vi "Dipper Fridge Resistance Measurement 1.2.vi"() -> ()   [LabVIEW 2011]
uses:
  <vilib>/express/express arith-compare/Formula/XNode/ExpressFormulaBlockNode.xnode
panel:
  in  "Timer":bool caption="Reset"
  out "Time Elapsed":string
  out "Output Power":dbl[unit]
  out "Heater Power (%)":string
  in  "Save":bool
  out "var":i32
  in  "error in (no error) 2":errorcluster
  in  "Output Range":string(combo)
  in  "Heater Power (%)":dbl caption="y"
  out "Heater Type (in Ohm)":string
  out "Heater Current (in %)":string
  out "Heater":bool
  in  "Heater":bool
  out "Boolean":bool
  in  "Power":bool
  in  "Date format (0)":enum16{"short", "long", "abbreviated"}(ring)
  out "Sample (Lakeshore)":cluster{dbl[], dbl[unit][]}(graph)
  out "Thermometer A":cluster{dbl[], dbl[unit][]}(graph)
  out "size (in bytes)":i64
  out "Thermometer (Ge17035)":cluster{dbl[], dbl[]}(graph)
  out "Warning":string="Can't be smaller than 1 s"
  in  "File Path":path
  out "current time":timestamp
  out "Number of Data points":i32
  in  "Time delay":u32=500 min=500 max=10000
  in  "error in (no error)":errorcluster
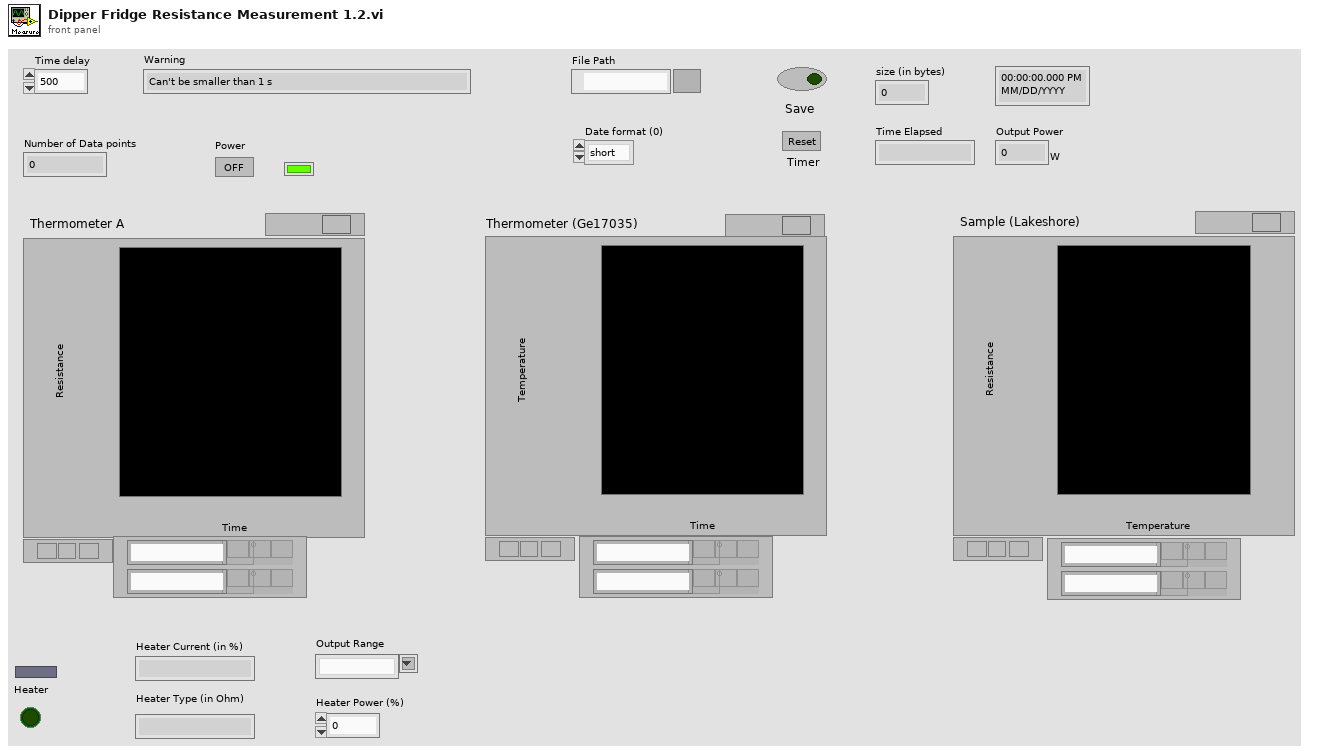
[diagram p1: front panel]
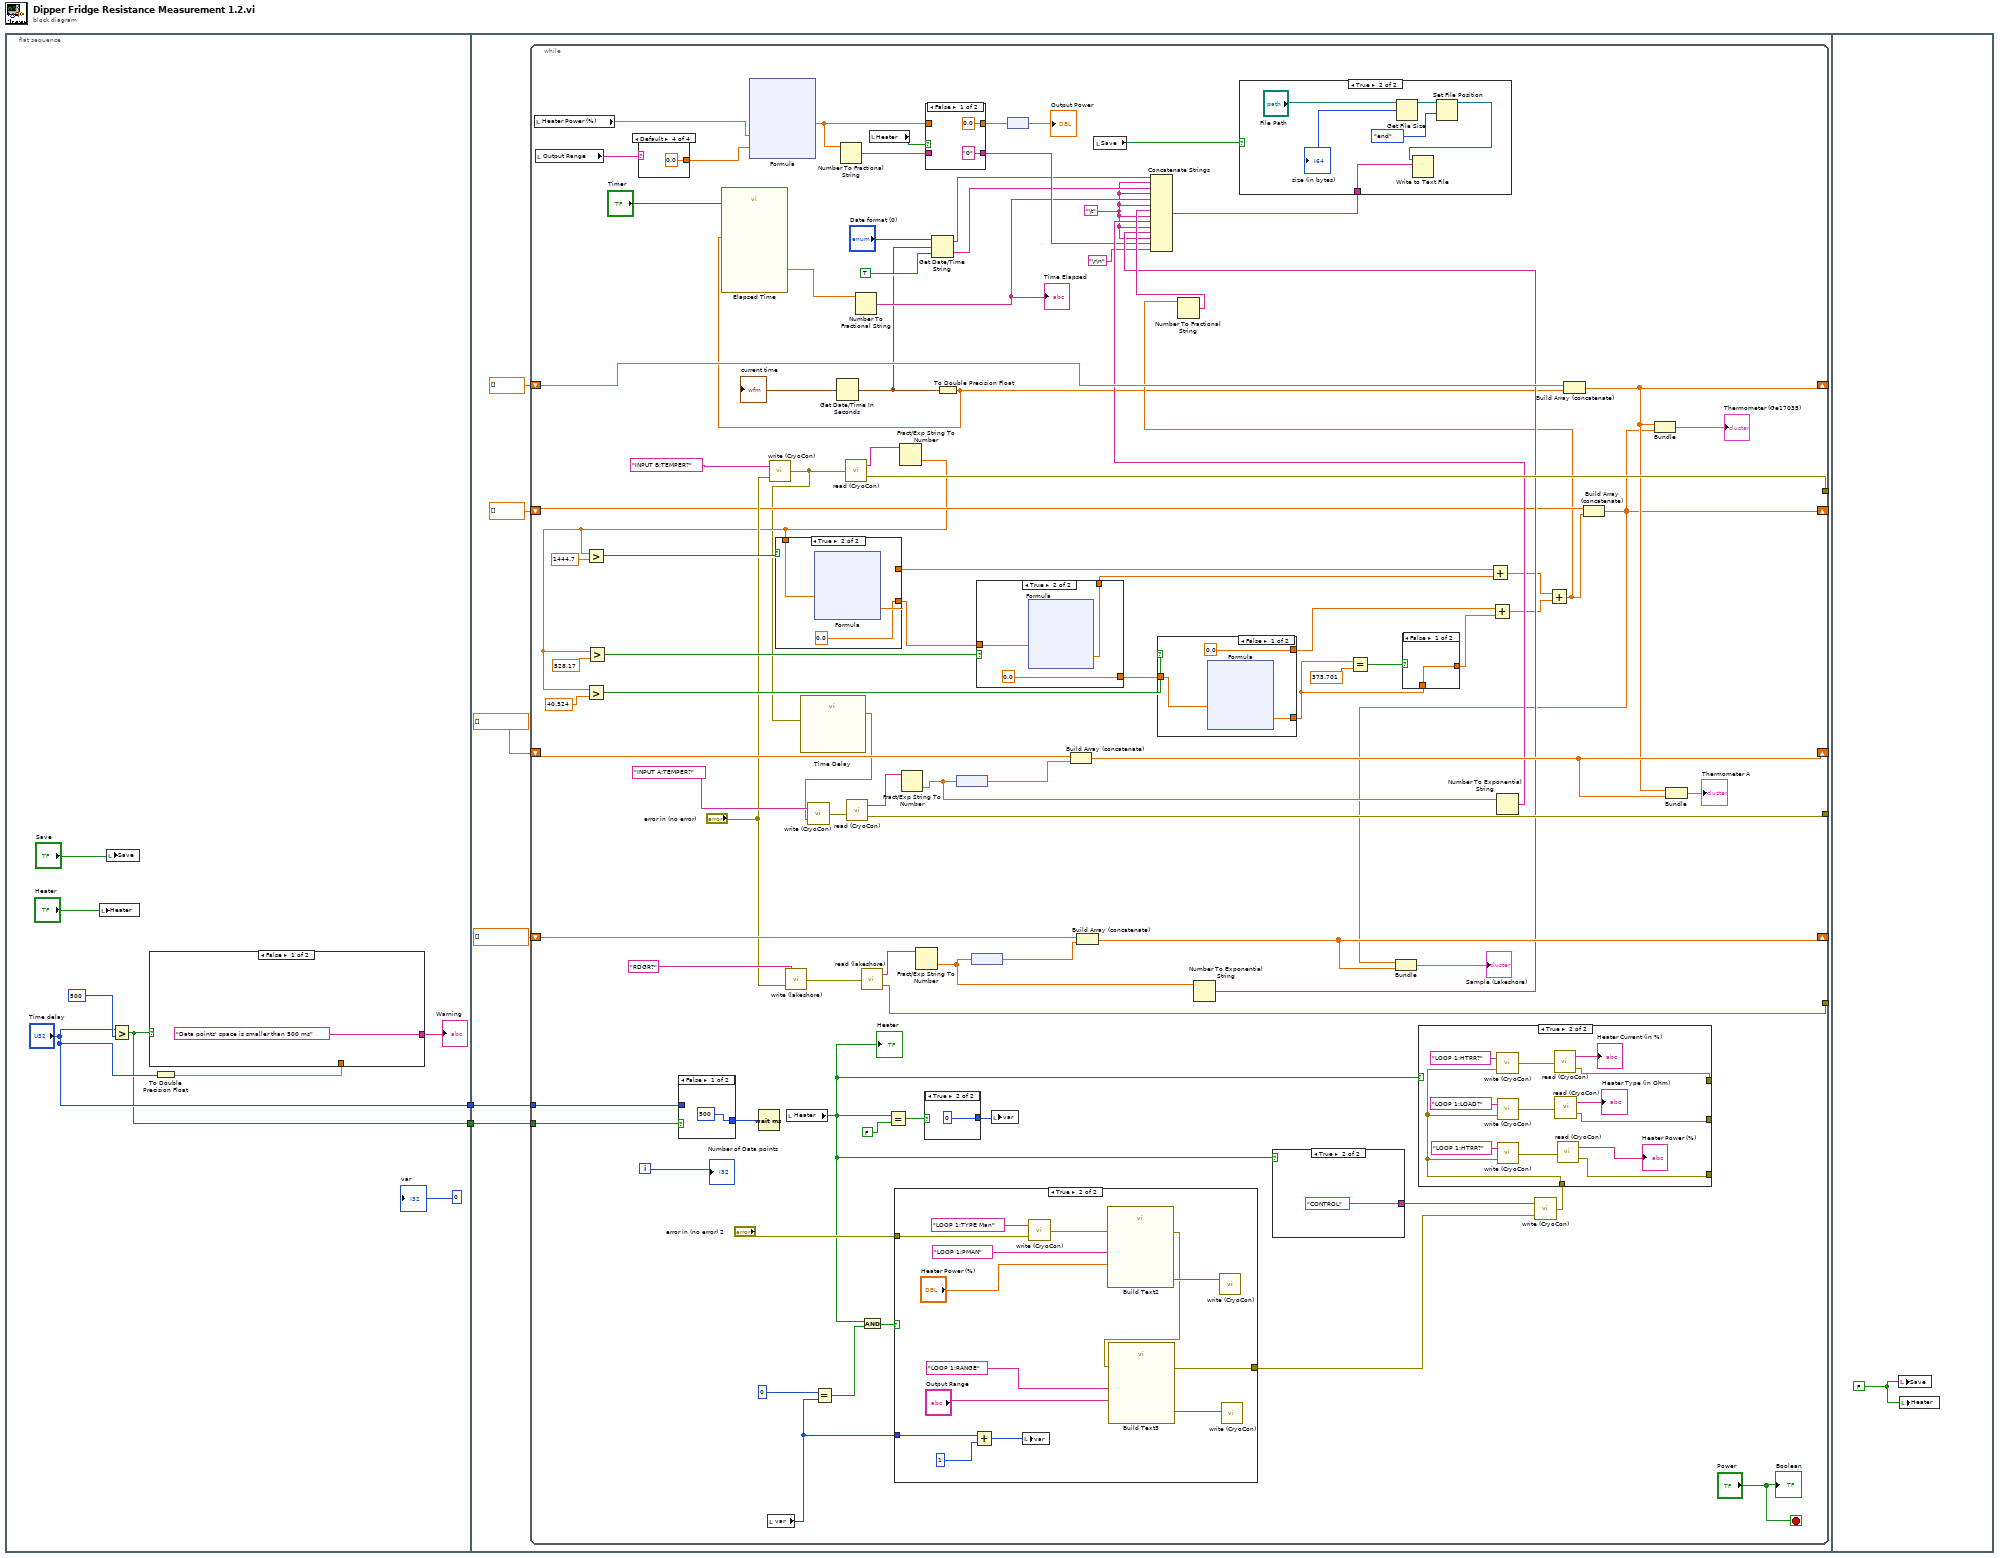
[diagram p0: block diagram]
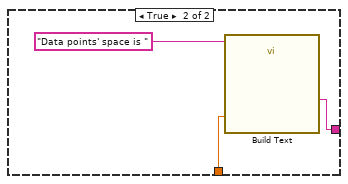
[diagram p2: hidden frame]
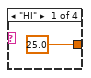
[diagram p4: hidden frame]
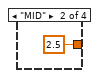
[diagram p5: hidden frame]
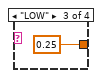
[diagram p6: hidden frame]
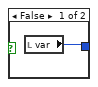
[diagram p7: hidden frame]
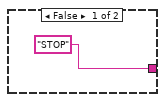
[diagram p10: hidden frame]
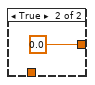
[diagram p11: hidden frame]
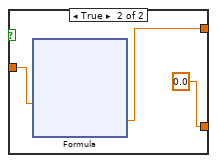
[diagram p12: hidden frame]
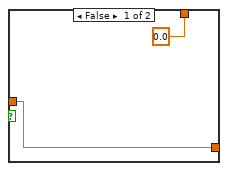
[diagram p13: hidden frame]
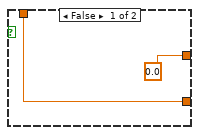
[diagram p14: hidden frame]
diagram:
  n1 = flat-sequence {
    tunnel: ["Time delay"] -> w2
    tunnel: [w5] -> w1
    tunnel: w2 -> [w20]
    tunnel: w1 -> [w19]
    frame #0 {
      n2 = local write "Heater"("Heater") -> ()
      n3 = local write "Save"("Save") -> ()
      n4 = Greater?(x="Time delay", y=u32 500 ("x")) -> (0:w5:bool)
      n5 = To Double Precision Float(number="Time delay") -> (double precision float=w7:dbl)
      n6 = case shown="False" w5 {
        tunnel: w7 -> [_ w12]
        tunnel: ["Data points' space is smaller than 500 ms" w14] -> w8
        frame False {
        }
        frame True {
          n7 = call "Build Text"("Beginning Text"="Data points' space is ", "Y"=w12) -> ("Result"=w14:string)  [unwired: 12 in, 1 out]
        }
      }
      "Warning" <- w8
      "var" <- 0 ("var")
    }
    frame #1 {
      n8 = while {
        tunnel: [w107] -> _
        tunnel: [w106] -> _
        tunnel: [w102] -> _
        shift-right: [w86] -> _
        shift-left: dbl[] [] -> [w97]
        tunnel: w20 -> [w96]
        tunnel: w19 -> [w95]
        shift-right: [w90] -> _
        shift-left: dbl[unit][] [] -> [w91]
        shift-right: [w87] -> _
        shift-left: dbl[unit][] [] -> [w88]
        shift-right: [w67] -> _
        shift-left: dbl[] [] -> [w70]
        i -> [w99]
        stop <- "Power" stop-if-true
        w21 = "\t"
        n9 = local read "Heater Power (%)"() -> (w41:dbl)
        n10 = local read "Output Range"() -> (w39:string)
        n11 = case shown="Default" w39 {
          tunnel: [25.0 ("X2") 2.5 ("X2") 0.25 ("X2") 0.0 ("X2")] -> w40
          frame "HI" {
          }
          frame "MID" {
          }
          frame "LOW" {
          }
          frame Default {
          }
        }
        n12 = case shown="False" w95 {
          tunnel: w96 -> [_ w213]
          tunnel: [500 w213] -> w94
          frame False {
          }
          frame True {
          }
        }
        n13 = xnode "Formula"("X1"=w41, "X2"=w40) -> ("Result"=w33:dbl)  [unwired: 1 in, 1 out]
        n14 = Wait (ms)(milliseconds to wait=w94) -> ()  [unwired: 1 out]
        n15 = local read "var"() -> (w51:i32)
        n16 = call "write (CryoCon).vi"("error in (no error)"="error in (no error)", "write buffer"="INPUT B:TEMPER?") -> ("error out"=w30:errorcluster)
        n17 = call "write (lakeshore).vi"("error in (no error)"="error in (no error)", "write buffer"="RDGR?") -> ("error out"=w101:errorcluster)
        n18 = local read "Heater"() -> (w42:bool)
        "Heater" <- w42
        n19 = call "Time Delay"("error in (no error)"=w30) -> ("error out"=w29:errorcluster)  [unwired: 10 in]
        n20 = call "write (CryoCon).vi"("error in (no error)"=w29, "write buffer"="INPUT A:TEMPER?") -> ("error out"=w108:errorcluster)
        n21 = Equal?(x=0, y=w51) -> (x = y?=w49:bool)
        n22 = Get Date/Time In Seconds() -> (seconds since 1Jan1904=w27:timestamp)
        "current time" <- w27
        n23 = Number To Fractional String(number=w33) -> (F-format string=w37:string)  [unwired: 3 in]
        n24 = call "read (CryoCon).vi"("error in (no error)"=w30) -> ("read buffer"=w104:string, "error out"=w106:errorcluster)
        n25 = call "read (CryoCon).vi"("error in (no error)"=w108) -> ("read buffer"=w105:string, "error out"=w107:errorcluster)
        n26 = call "read (lakeshore).vi"("error in (no error)"=w101) -> ("read buffer"=w103:string, "error out"=w102:errorcluster)
        n27 = And(x=w42, y=w49) -> (x .and. y?=w48:bool)
        n28 = local read "Heater"() -> (w35:bool)
        n29 = Equal?(x=w42, y=FALSE ("Heater")) -> (x = y?=w44:bool)
        n30 = case shown="True" w48 {
          tunnel: [w131 w139] -> w47
          tunnel: "error in (no error) 2" -> [w131 w135]
          tunnel: w51 -> [_ w138]
          frame False {
          }
          frame True {
            n31 = Add(x=w138, y=1) -> (x+y=w136:i32)
            n32 = local write "var"(w136) -> ()
            n33 = call "write (CryoCon).vi"("error in (no error)"=w135, "write buffer"="LOOP 1:TYPE Man") -> ("error out"=w134:errorcluster)
            n34 = call "Build Text2"("x"="LOOP 1:PMAN" ("write buffer"), "y"="Heater Power (%)", "error in (no error)"=w134) -> ("Result"=w144:string, "error out"=w140:errorcluster)  [unwired: 11 in]
            n35 = call "Build Text3"("x"="LOOP 1:RANGE" ("write buffer"), "y"="Output Range", "error in (no error)"=w140) -> ("Result"=w141:string, "error out"=w139:errorcluster)  [unwired: 11 in]
            n36 = call "write (CryoCon).vi"("write buffer"=w144) -> ()  [unwired: 1 in, 1 out]
            n37 = call "write (CryoCon).vi"("write buffer"=w141) -> ()  [unwired: 1 in, 1 out]
          }
        }
        n38 = Fract/Exp String To Number(string=w104) -> (number=w31:dbl)  [unwired: 3 in, 1 out]
        n39 = Greater?(x=w31, y=1444.7) -> (0:w78:bool)
        n40 = Greater?(x=w31, y=40.524) -> (0:w75:bool)
        n41 = Greater?(x=w31, y=528.17) -> (0:w77:bool)
        n42 = case shown="True" w78 {
          tunnel: w31 -> [w199 w203]
          tunnel: [0.0 w202] -> w64
          tunnel: [w199 0.0] -> w61
          frame False {
          }
          frame True {
            n43 = xnode "Formula"("X1"=w203) -> ("Result"=w202:dbl)  [unwired: 1 in, 1 out]
          }
        }
        n44 = Fract/Exp String To Number(string=w105) -> (number=w84:dbl)  [unwired: 3 in, 1 out]
        n45 = Fract/Exp String To Number(string=w103) -> (number=w83:dbl)  [unwired: 3 in, 1 out]
        n46 = case shown="True" w44 {
          tunnel: [w119 0] -> w43
          frame False {
            n47 = local read "var"() -> (w119:i32)
          }
          frame True {
          }
        }
        n48 = case shown="False" w35 {
          tunnel: w37 -> [_ w114]
          tunnel: ["0" w114] -> w36
          tunnel: w33 -> [_ w113]
          tunnel: [0.0 ("Result") w113] -> w32
          frame False {
          }
          frame True {
          }
        }
        n49 = Get Date/Time String(date format (0)="Date format (0)", seconds (now)=w27, want seconds? (F)=TRUE) -> (date string=w22:string, time string=w23:string)
        n50 = To Double Precision Float(number=w27) -> (double precision float=w25:dbl)
        n51 = call "Elapsed Time"("Reset"="Timer", "Set Start Time (s)"=w25) -> ("Elapsed Time (s)"=w26:dbl)  [unwired: 10 in, 7 out]
        n52 = Number To Fractional String(number=w26) -> (F-format string=w28:string)  [unwired: 3 in]
        "Time Elapsed" <- w28
        n53 = node(w84) -> (w92:dbl[unit])
        n54 = node(w83) -> (w69:dbl[unit])
        n55 = case shown="True" w77 {
          tunnel: [0.0 w190] -> w63
          tunnel: w61 -> [w186 w189]
          tunnel: [w186 0.0] -> w60
          frame False {
          }
          frame True {
            n56 = xnode "Formula"("X2"=w189) -> ("Result"=w190:dbl)  [unwired: 1 in, 1 out]
          }
        }
        n57 = local write "var"(w43) -> ()
        n58 = node(w32) -> (→"Output Power":dbl[unit])
        n59 = Build Array (concatenate)(w91, w92) -> (w90:dbl[unit][])
        n60 = Build Array (concatenate)(w88, w69) -> (w87:dbl[unit][])
        n61 = local read "Save"() -> (w46:bool)
        n62 = case shown="False" w75 {
          tunnel: [0.0 w177] -> w62
          tunnel: [w165 0.0] -> w56
          tunnel: w60 -> [w164 w175]
          frame False {
            n63 = xnode "Formula"("X4"=w164) -> ("Result"=w165:dbl)  [unwired: 1 in, 1 out]
          }
          frame True {
            n64 = xnode "Formula"("X3"=w175) -> ("Result"=w177:dbl)  [unwired: 1 in, 1 out]
          }
        }
        n65 = Number To Exponential String(number=w83) -> (E-format string=w80:string)  [unwired: 3 in]
        n66 = case shown="True" w42 {
          tunnel: ["STOP" ("write buffer") "CONTROL" ("write buffer")] -> w54
          frame False {
          }
          frame True {
          }
        }
        n67 = Equal?(x=w56, y=375.701) -> (x = y?=w59:bool)
        n68 = case shown="False" w59 {
          tunnel: [w162 0.0 ("y")] -> w57
          tunnel: w56 -> [w162 _]
          frame False {
          }
          frame True {
          }
        }
        n69 = Add(x=w64, y=w63) -> (x+y=w72:dbl)
        n70 = Add(x=w62, y=w57) -> (x+y=w71:dbl)
        n71 = Number To Exponential String(number=w84) -> (E-format string=w81:string)  [unwired: 3 in]
        n72 = call "write (CryoCon).vi"("error in (no error)"=w47, "write buffer"=w54) -> ("error out"=w53:errorcluster)
        n73 = case shown="True" w42 {
          tunnel: [w146 w153] -> _
          tunnel: [w146 w152] -> _
          tunnel: w53 -> [w146 w151]
          tunnel: [w146 w150] -> _
          frame False {
          }
          frame True {
            n74 = call "write (CryoCon).vi"("error in (no error)"=w151, "write buffer"="LOOP 1:HTRR?") -> ("error out"=w159:errorcluster)
            n75 = call "write (CryoCon).vi"("error in (no error)"=w151, "write buffer"="LOOP 1:LOAD?") -> ("error out"=w156:errorcluster)
            n76 = call "write (CryoCon).vi"("error in (no error)"=w151, "write buffer"="LOOP 1:HTRR?") -> ("error out"=w149:errorcluster)
            n77 = call "read (CryoCon).vi"("error in (no error)"=w159) -> ("read buffer"=→"Heater Current (in %)":string, "error out"=w153:errorcluster)
            n78 = call "read (CryoCon).vi"("error in (no error)"=w156) -> ("read buffer"=→"Heater Type (in Ohm)":string, "error out"=w152:errorcluster)
            n79 = call "read (CryoCon).vi"("error in (no error)"=w149) -> ("read buffer"=→"Heater Power (%)":string, "error out"=w150:errorcluster)
          }
        }
        n80 = Add(x=w72, y=w71) -> (x+y=w55:dbl)
        n81 = Number To Fractional String(number=w55) -> (F-format string=w82:string)  [unwired: 3 in]
        n82 = Concatenate Strings(w22, w21, w23, w21, w28, w21, w82, w21, w81, w21, w80, w21, w36, "\r\n") -> (w93:string)
        n83 = case shown="True" w46 {
          tunnel: w93 -> [_ w219]
          frame False {
          }
          frame True {
            n84 = Get File Size(file="File Path") -> (refnum out=w217:refnum<file>, size (in bytes)=→"size (in bytes)":i64)  [unwired: 1 in, 1 out]
            n85 = Set File Position(refnum=w217, from (0:start)=enum16{"start", "end", "current"}."end") -> (refnum out=w216:refnum<file>)  [unwired: 2 in, 1 out]
            n86 = Write to Text File(file (use dialog)=w216, text=w219) -> ()  [unwired: 2 in, 3 out]
          }
        }
        n87 = Build Array (concatenate)(w97, w25) -> (w86:dbl[])
        n88 = Build Array (concatenate)(w70, w55) -> (w67:dbl[])
        n89 = Bundle(w67, w87) -> (→"Sample (Lakeshore)":cluster{dbl[], dbl[unit][]})  [unwired: 1 in]
        n90 = Bundle(w86, w67) -> (→"Thermometer (Ge17035)":cluster{dbl[], dbl[]})  [unwired: 1 in]
        n91 = Bundle(w86, w90) -> (→"Thermometer A":cluster{dbl[], dbl[unit][]})  [unwired: 1 in]
        "Number of Data points" <- w99
        "Boolean" <- "Power"
      }
    }
    frame #2 {
      w220 = FALSE ("Save")
      n92 = local write "Save"(w220) -> ()
      n93 = local write "Heater"(w220) -> ()
    }
  }
